vi "Auth Async.vi"(4 "Failed Response":refnum<class "Response.lvclass">, 6 "Complete Response":refnum<class "Response.lvclass">, 9 "Timeout S":dbl=60.0, 10 "Async Authorization":refnum<class "Async Authorization.lvclass">, 11 "OAuth2 in":refnum<class "OAuth2.lvclass">) -> ()   [LabVIEW 2020, in "OAuth2.lvlib" / "OAuth2.lvclass"]
uses:
  OAuth2.lvclass
  Async Authorization/Async Authorization.lvclass
  HTTP Utils/Response/Response.lvclass
  Async Auth State.ctl
  OAuth2.lvclass/OAuth2.ctl
  <vilib>/Platform/browser.llb/Open URL in Default Browser (string).vi
  <vilib>/Utility/error.llb/Error Cluster From Error Code.vi
  <vilib>/httpClient/POSTBuffer.vi
  <vilib>/ErrorRing/Error Ring.xnode
  OAuth2.lvlib
  HTTP Utils/Request/Request.lvclass
  Request/Request.lvclass
  <vilib>/httpClient/LabVIEWHTTPClient.lvlib
panel:
  out "Request URL":string
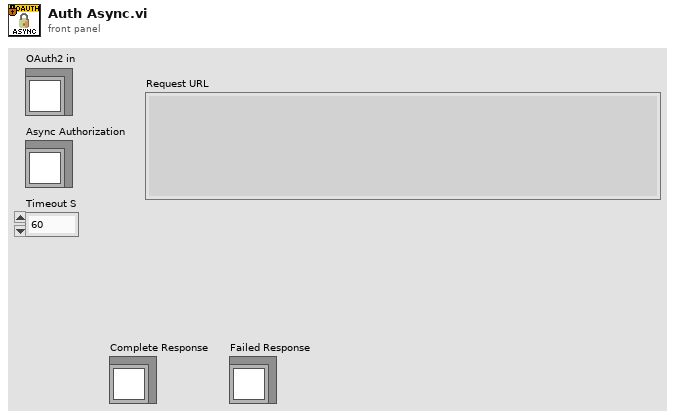
[diagram p1: front panel]
types:
  T1 = typedef "OAuth2.lvlib/Async Auth State.ctl" = enum16{"Idle", "Request", "WaitAuth", "GetToken", "RefreshToken", "Complete", "Failed"}
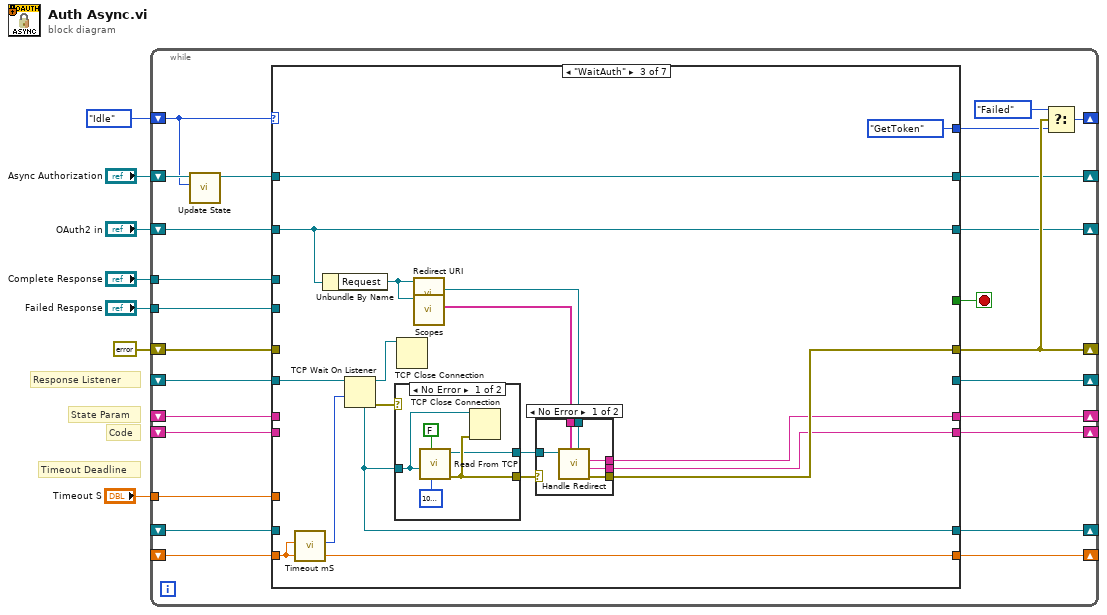
[diagram p0: block diagram]
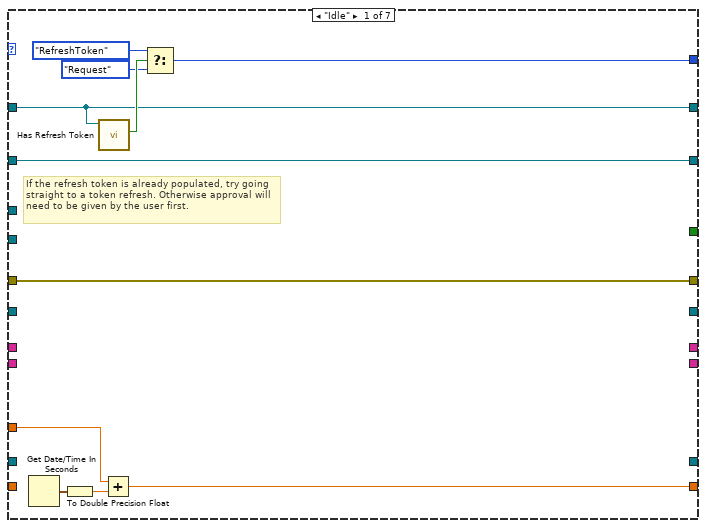
[diagram p2: hidden frame]
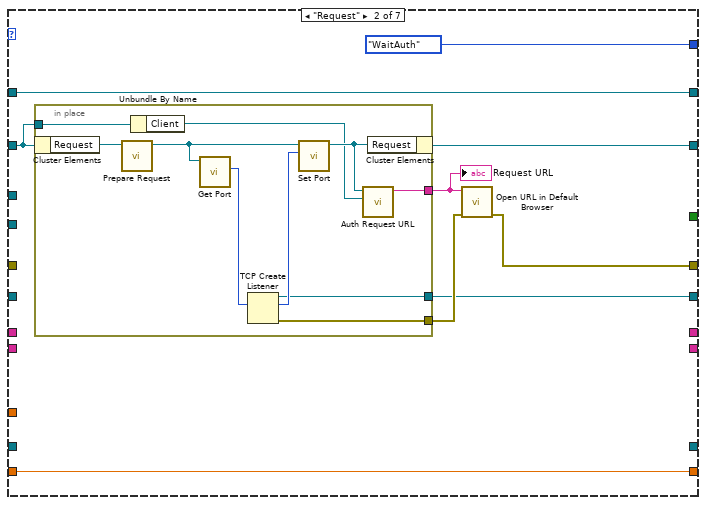
[diagram p3: hidden frame]
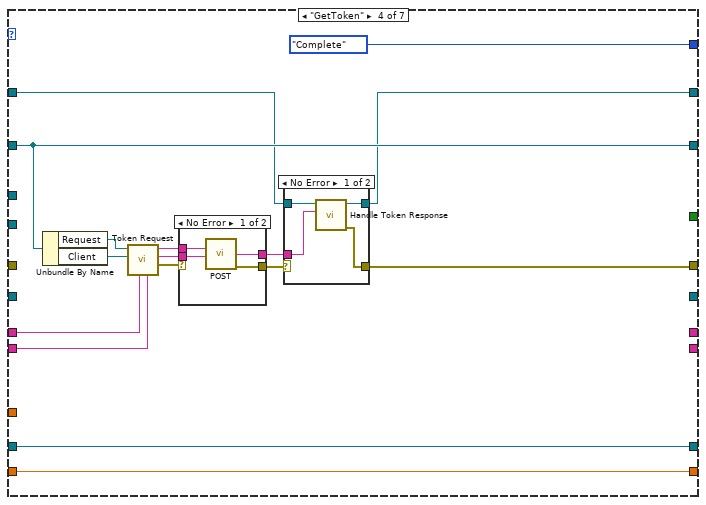
[diagram p6: hidden frame]
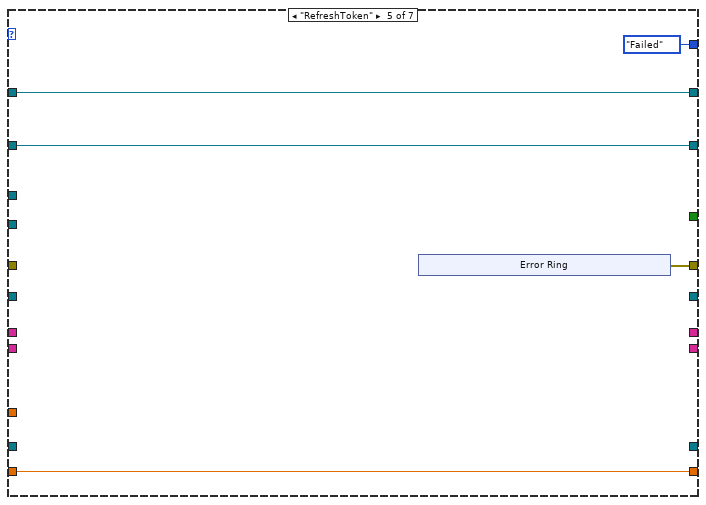
[diagram p9: hidden frame]
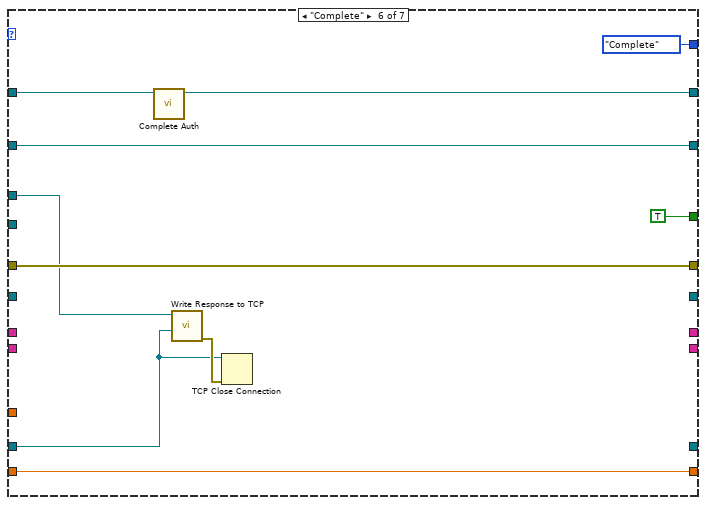
[diagram p10: hidden frame]
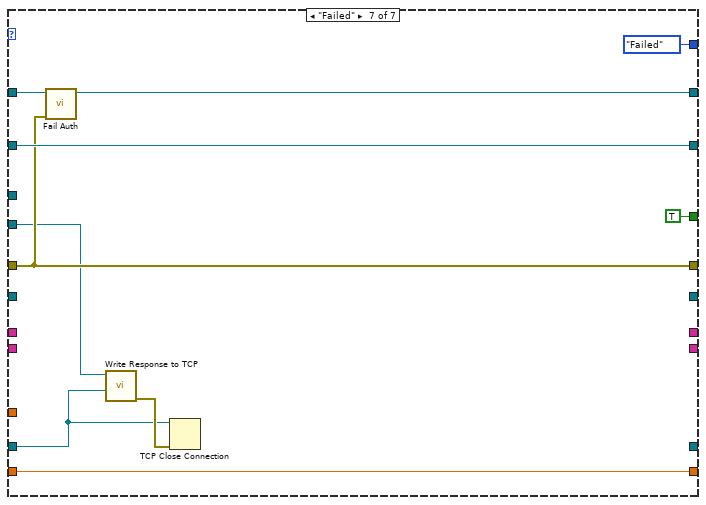
[diagram p11: hidden frame]
diagram:
  # "Timeout Deadline"
  # "Code"
  # "State Param"
  # "Response Listener"
  n1 = while {
    shift-right: [w16] -> _
    shift-left: Async_Auth_State."Idle" ("State") -> [w26]
    shift-right: [w30] -> _
    shift-left: "OAuth2 in" -> [w31]
    shift-right: [w25] -> _
    shift-left: _ -> [w29]
    shift-right: [w24] -> _
    shift-left: _ -> [w22]
    shift-right: [w23] -> _
    shift-left: _ -> [w21]
    tunnel: "Timeout S" -> [w20]
    shift-right: [w19] -> _
    shift-left: _ -> [w18]
    shift-right: [w32] -> _
    shift-left: errorcluster {"status"=FALSE, "code"=0, "source"=""} ("error out") -> [w17]
    shift-right: [w13] -> _
    shift-left: "Async Authorization" -> [w28]
    tunnel: "Complete Response" -> [w11]
    tunnel: "Failed Response" -> [w10]
    shift-right: [w9] -> _
    shift-left: _ -> [w8]
    stop <- w12 stop-if-true
    n2 = call "Update State.vi"("Async Auth State"=w26, "Async Authorization in"=w28) -> ("Async Authorization out"=w27:refnum<class "Async Authorization.lvclass">)  [unwired: 9 in]
    n3 = case shown="\"WaitAuth\"" w26 {
      tunnel: w31 -> [w43 w50 w66 w108 w124 w132 w147]
      tunnel: [w43 w48 w66 w108 w124 w132 w147] -> w30
      tunnel: w29 -> [_ _ w78 _ _ _ _]
      tunnel: w27 -> [w34 w44 w73 w94 w122 w133 w145]
      tunnel: [_ w51 _ _ _ _ _] -> w25
      tunnel: [_ _ w68 _ _ _ _] -> w24
      tunnel: [_ _ w67 _ _ _ _] -> w23
      tunnel: w22 -> [_ _ _ w105 _ _ _]
      tunnel: w21 -> [_ _ _ w104 _ _ _]
      tunnel: w20 -> [w37 _ _ _ _ _ _]
      tunnel: [w36 w46 w77 w100 w123 w137 w146] -> w19
      tunnel: w18 -> [_ w46 w77 w100 w123 w137 w146]
      tunnel: [w33 w47 w69 w97 w120 w135 w141] -> w32
      tunnel: w17 -> [w33 _ _ _ _ w135 w141]
      tunnel: [w35 Async_Auth_State."WaitAuth" ("State") Async_Auth_State."GetToken" ("f") Async_Auth_State."Complete" ("f") Async_Auth_State."Failed" ("f") Async_Auth_State."Complete" ("f") Async_Auth_State."Failed" ("f")] -> w14
      tunnel: [w34 w44 w73 w95 w122 w131 w144] -> w13
      tunnel: [_ _ _ _ _ TRUE TRUE] -> w12
      tunnel: w11 -> [_ _ _ _ _ w129 _]
      tunnel: w10 -> [_ _ _ _ _ _ w140]
      tunnel: [_ _ w72 w93 _ _ _] -> w9
      tunnel: w8 -> [_ _ _ w93 _ w130 w139]
      frame "Idle" {
        # "If the refresh token is already populated, try going straight to a token refresh. Otherwise approval will need to be given by the user first."
        n4 = Get Date/Time In Seconds() -> (seconds since 1Jan1904=w39:timestamp)
        n5 = To Double Precision Float(number=w39) -> (double precision float=w38:dbl)
        n6 = call "Has Refresh Token.vi"("Async Authorization in"=w34) -> ("Has Refresh Token"=w42:bool)  [unwired: 10 in]
        n7 = Add(x=w37, y=w38) -> (x+y=w36:dbl)
        n8 = Select(t=Async_Auth_State."RefreshToken" ("State"), s=w42, f=Async_Auth_State."Request") -> (s? t:f=w35:T1)
      }
      frame "Request" {
        n9 = in-place {
          in-place-border: [w60] -> w51
          in-place-border: w50 -> [w59]
          in-place-border: [w56] -> w49
          in-place-border: [w55] -> w52
          n10 = in-place-cluster #1(w50) -> ("Request"=w54:refnum<class "Request.lvclass">)
          n11 = call "Prepare Request.vi"("Request in"=w54) -> ("Request out"=w53:refnum<class "Request.lvclass">)  [unwired: 10 in]
          n12 = Unbundle By Name(w59) -> ("Client"=w57:refnum<class "Client.lvclass">)
          n13 = call "Get Port.vi"("Request in"=w53) -> ("Port"=w62:u16)  [unwired: 10 in]
          n14 = TCP Create Listener(10:w62) -> (0:w55:errorcluster, 2:w61:u16, 3:w60:refnum<k5>)  [unwired: 4 in]
          n15 = call "Set Port.vi"("Port"=w61, "Request in"=w53) -> ("Request out"=w58:refnum<class "Request.lvclass">)  [unwired: 9 in]
          n16 = call "Auth Request URL.vi"("Client"=w57, "Request in"=w58) -> ("Request URL"=w56:string)  [unwired: 9 in]
          n17 = in-place-cluster #1("Request"=w58) -> (w48:refnum<class "OAuth2.lvclass">)
        }
        "Request URL" <- w49
        n18 = call-poly <vilib>:"Open URL in Default Browser.vi"("error in (no error)"=w52, "URL"=w49) -> ("error out"=w47:errorcluster)  [unwired: 4 in, 1 out]
      }
      frame "WaitAuth" {
        n19 = call "Timeout mS.vi"("Deadline"=w77) -> ("Timeout mS"=w76:i32)  [unwired: 10 in]
        n20 = Unbundle By Name(w66) -> ("Request"=w64:refnum<class "Request.lvclass">)
        n21 = TCP Wait On Listener(9:w76, 11:w78) -> (0:w79:errorcluster, 3:w75:refnum<k5>, 4:w72:refnum<k5>)  [unwired: 2 in, 2 out]
        n22 = case shown="No Error" w79 {
          selector: w79 -> [_ w92]
          tunnel: w72 -> [w87 _]
          tunnel: [w91 w92] -> w71
          tunnel: [w88 _] -> w70
          frame No Error {
            n23 = call "Read From TCP.vi"("Max Size (50MB)"=u64 1000000, "Uploads as Files? (T)"=FALSE, "TCP Connection"=w87) -> ("error out"=w91:errorcluster, "Request out"=w88:refnum<class "Request.lvclass">)  [unwired: 7 in]
            n24 = TCP Close Connection(connection ID=w87, error in (no error)=w91) -> ()  [unwired: 1 in, 2 out]
          }
          frame Error {
          }
        }
        n25 = TCP Close Connection(connection ID=w75) -> ()  [unwired: 2 in, 2 out]
        n26 = call "Redirect URI.vi"("Request in"=w64) -> ("Redirect URI"=w63:refnum<class "URI.lvclass">)  [unwired: 10 in]
        n27 = call "Scopes.vi"("Request in"=w64) -> ("Scopes"=w65:string[])  [unwired: 10 in]
        n28 = case shown="No Error" w71 {
          selector: w71 -> [_ w86]
          tunnel: w70 -> [w85 _]
          tunnel: [w84 w86] -> w69
          tunnel: [w83 _] -> w68
          tunnel: [w82 _] -> w67
          tunnel: w65 -> [w81 _]
          tunnel: w63 -> [w80 _]
          frame No Error {
            n29 = call "Handle Redirect.vi"("Redirect URI"=w80, "Requested Scopes"=w81, "Request in"=w85) -> ("error out"=w84:errorcluster, "Code"=w82:string, "State Param"=w83:string)  [unwired: 6 in]
          }
          frame Error {
          }
        }
      }
      frame "GetToken" {
        n30 = Unbundle By Name(w108) -> ("Request"=w107:refnum<class "Request.lvclass">, "Client"=w106:refnum<class "Client.lvclass">)
        n31 = call "Token Request.vi"("Code"=w104, "State"=w105, "Client"=w106, "Request in"=w107) -> ("error out"=w103:errorcluster, "POST Buffer"=w102:string, "Request URL"=w101:string)  [unwired: 5 in]
        n32 = case shown="No Error" w103 {
          selector: w103 -> [_ w119]
          tunnel: w102 -> [w117 _]
          tunnel: w101 -> [w118 _]
          tunnel: [w116 w119] -> w99
          tunnel: [w115 _] -> w98
          frame No Error {
            n33 = call-poly <vilib>:"POST.vi"("url"=w118, "buffer"=w117) -> ("body"=w115:string, "error out"=w116:errorcluster)  [unwired: 10 in, 2 out]
          }
          frame Error {
          }
        }
        n34 = case shown="No Error" w99 {
          selector: w99 -> [_ w114]
          tunnel: w98 -> [w111 _]
          tunnel: w94 -> [w112 w113]
          tunnel: [w110 w114] -> w97
          tunnel: [w109 w113] -> w95
          frame No Error {
            n35 = call "Handle Token Response.vi"("Response Body"=w111, "Async Authorization in"=w112) -> ("error out"=w110:errorcluster, "Asyn Authorization out"=w109:refnum<class "Async Authorization.lvclass">)  [unwired: 8 in]
          }
          frame Error {
          }
        }
      }
      frame "RefreshToken" {
        n36 = xnode "Error Ring"() -> ("error out"=w120:errorcluster)
      }
      frame "Complete" {
        (unwired) TRUE
        n37 = call "Complete Auth.vi"("Async Authorization in"=w133) -> ("Async Authorization out"=w131:refnum<class "Async Authorization.lvclass">)  [unwired: 9 in, 1 out]
        n38 = call "Write Response to TCP.vi"("TCP Connection"=w130, "Response in"=w129) -> ("error out"=w138:errorcluster)  [unwired: 8 in, 1 out]
        n39 = TCP Close Connection(connection ID=w130, error in (no error)=w138) -> ()  [unwired: 1 in, 2 out]
      }
      frame "Failed" {
        (unwired) TRUE
        n40 = call "Fail Auth.vi"("error in (no error)"=w141, "Async Authorization in"=w145) -> ("Async Authorization out"=w144:refnum<class "Async Authorization.lvclass">)  [unwired: 8 in, 1 out]
        n41 = call "Write Response to TCP.vi"("TCP Connection"=w139, "Response in"=w140) -> ("error out"=w148:errorcluster)  [unwired: 8 in, 1 out]
        n42 = TCP Close Connection(connection ID=w139, error in (no error)=w148) -> ()  [unwired: 1 in, 2 out]
      }
    }
    n43 = Select(t=Async_Auth_State."Failed" ("State"), s=w32, f=w14) -> (s? t:f=w16:T1)
  }
